vi "Connect and Disconnect.vi"   [LabVIEW 2020]
uses:
  Nominal Client/Nominal Client.lvclass/Nominal Client.ctl
  5de6f169-3779-4eeb-a6de-3f17e36a8f54.vi
  b8c625b9-7f41-4907-b61e-90a3f4e11cd5.vi
  ac5b66b4-fbaa-40ae-a2c1-6e117ed88ff8.vi
  Nominal Client/private_data.set.vi
  <vilib>/Utility/error.llb/Error Cluster From Error Code.vi
  submodules/reqwest-labview/lv-src/reqwest/create.vi
  <vilib>/Utility/file.llb/Application Directory.vi
  Nominal Client/Nominal Client.lvclass
  nominal types/workspace/workspace.lvclass
  submodules/reqwest-labview/lv-src/reqwest/reqwest.lvclass
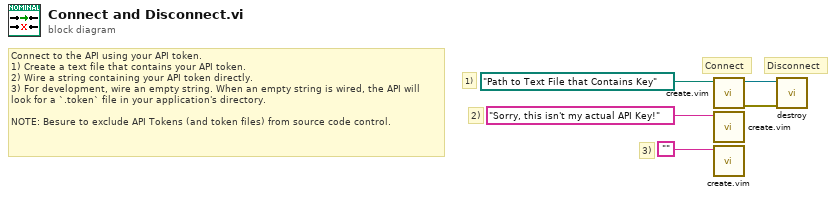
[diagram p0: block diagram]
diagram:
  # "Disconnect"
  # "Connect"
  # "3)"
  # "2)"
  # "1)"
  # "Connect to the API using your API token.\n1) Create a text file that contains your API token.\n2) Wire a string containing your API token directly.\n3) For development, wire an empty string. When an empty string is wired, the API will look for a `.token` file in your application's directory.\n\nNOTE: Besure to exclude API Tokens (and token files) from source code control."
  n1 = call "create.vim"("API Token (string or path)"=path "Path to Text File that Contains Key") -> ("error out"=w4:errorcluster, "Nominal Client"=w5:refnum<class "Nominal Client.lvclass">)  [unwired: 9 in]
  n2 = call "create.vim"("API Token (string or path)"="Sorry, this isn't my actual API Key!") -> ()  [unwired: 9 in, 2 out]
  n3 = call "create.vim"("API Token (string or path)"="") -> ()  [unwired: 9 in, 2 out]
  n4 = call "destroy.vi"("error in"=w4, "Nominal Client"=w5) -> ()  [unwired: 9 in, 1 out]
